vi "Calculate_Times.vi"(0 "Input Times":T1) -> (1 "Total Percent":dbl, 2 "Total String":string, 3 "Current Percent":dbl, 4 "Current String":string)   [LabVIEW 2011]
doc: "This VI uses a cluster input as a space-saving convenience. It simply converts the given inputs to \"Total Percent\", which indicates what percentage of the entire growth run has been completed; the \"Total String\", which is a string indicating the remaining time in the format of MM:SS; the \"Current Percent\", which indicates what percentage of the current event has been completed; and the \"Current String\", which indicates the remaining time of the current event in the format of MM:SS."
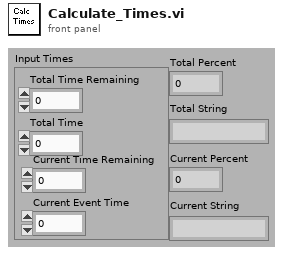
[diagram p1: front panel]
types:
  T1 = cluster{"Total Time Remaining":dbl, "Total Time":dbl, "Current Time Remaining":dbl, "Current Event Time":dbl}
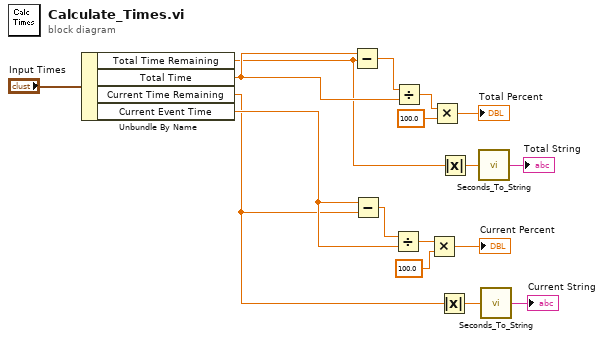
[diagram p0: block diagram]
diagram:
  n1 = Unbundle By Name("Input Times") -> ("Total Time Remaining"=w1:dbl, "Total Time"=w6:dbl, "Current Time Remaining"=w4:dbl, "Current Event Time"=w5:dbl)
  n2 = Subtract(x=w6, y=w1) -> (x-y=w8:dbl)
  n3 = Subtract(x=w5, y=w4) -> (x-y=w13:dbl)
  n4 = Divide(x=w13, y=w5) -> (x/y=w12:dbl)
  n5 = Divide(x=w8, y=w6) -> (x/y=w17:dbl)
  n6 = Multiply(x=w12, y=100.0) -> (x*y=→"Current Percent":dbl)
  n7 = Multiply(x=w17, y=100.0) -> (x*y=→"Total Percent":dbl)
  n8 = Absolute Value(x=w4) -> (abs(x)=w3:dbl)
  n9 = Absolute Value(x=w1) -> (abs(x)=w2:dbl)
  n10 = call "Seconds_To_String.vi"("Seconds"=w2) -> ("Output String"=→"Total String":string)
  n11 = call "Seconds_To_String.vi"("Seconds"=w3) -> ("Output String"=→"Current String":string)
